vi "Find All Zeroes Inner Part (VI).vi"(6 "data":variant, 7 "f(x)":T1, 8 "error in":i32, 9 "accuracy":dbl=1e-08 format="%.2e", 10 "algorithm":u16, 11 "X and Y values":cluster{"X Values":dbl[], "Y Values":dbl[]} {"Y Values" format="%.2f"; "X Values" format="%.2f"}) -> (0 "error out":i32, 2 "f(Zeroes)":dbl[](array[numeric]) format="%.2f", 3 "Zeroes":dbl[](array[numeric]) format="%.2f")   [LabVIEW 2010, in "NI_Gmath.lvlib"]
uses:
  NI_Gmath.lvlib
  functionRefnum.ctl
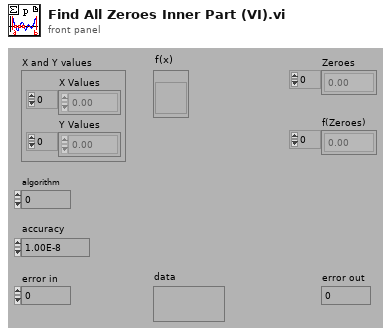
[diagram p1: front panel]
types:
  T1 = typedef "NI_Gmath.lvlib/functionRefnum.ctl" = refnum<vi>
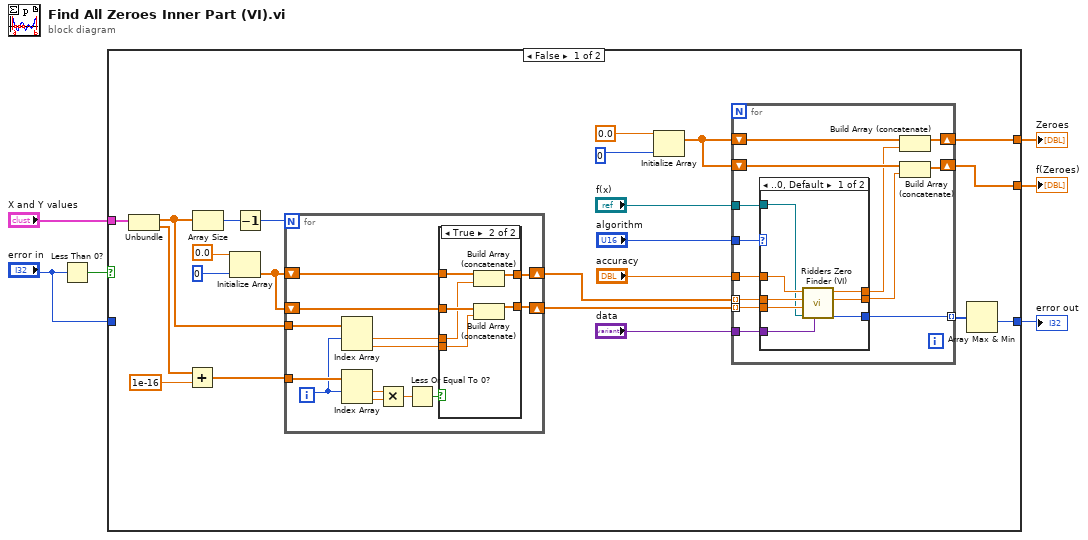
[diagram p0: block diagram]
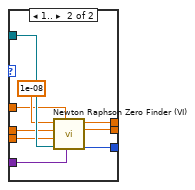
[diagram p2: hidden frame]
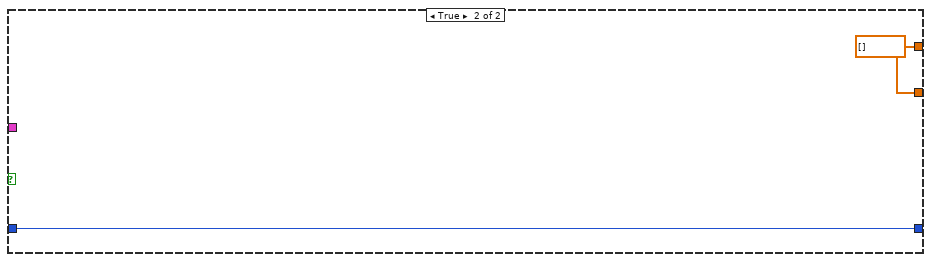
[diagram p4: hidden frame]
diagram:
  n1 = Less Than 0?(x="error in") -> (x < 0?=w2:bool)
  n2 = case shown="False" w2 {
    tunnel: "X and Y values" -> [w20 _]
    tunnel: [w11 w81] -> w5
    tunnel: [w10 w81] -> w4
    tunnel: [w9 w82] -> w3
    tunnel: "error in" -> [_ w82]
    frame False {
      n3 = Unbundle(w20) -> ("X Values"=w29:dbl[], "Y Values"=w23:dbl[])
      n4 = Add(x=w23, y=1e-16) -> (x+y=w25:dbl[])
      n5 = Array Size(array=w29) -> (size(s)=w21:i32)
      n6 = Initialize Array(0.0, 0) -> (w28:dbl[])
      n7 = Decrement(x=w21) -> (x-1=w22:i32)
      n8 = for {
        N: w22 -> [_]
        tunnel: w25 -> [w63]
        shift-right: [w69] -> w15
        shift-left: w28 -> [w70]
        shift-right: [w67] -> w14
        shift-left: w28 -> [w68]
        tunnel: w29 -> [w66]
        i -> [w60]
        n9 = Index Array(array=w66, index #1=w60) -> (element #1=w65:dbl, element #2=w64:dbl)  [unwired: 1 in]
        n10 = Index Array(array=w63, index #1=w60) -> (element #1=w62:dbl, element #2=w61:dbl)  [unwired: 1 in]
        n11 = Multiply(x=w62, y=w61) -> (x*y=w72:dbl)
        n12 = Less Or Equal To 0?(x=w72) -> (x <= 0?=w71:bool)
        n13 = case shown="True" w71 {
          tunnel: w70 -> [w74 w80]
          tunnel: [w74 w79] -> w69
          tunnel: w68 -> [w73 w78]
          tunnel: [w73 w77] -> w67
          tunnel: w65 -> [_ w76]
          tunnel: w64 -> [_ w75]
          frame False {
          }
          frame True {
            n14 = Build Array (concatenate)(w80, w76) -> (w79:dbl[])
            n15 = Build Array (concatenate)(w78, w75) -> (w77:dbl[])
          }
        }
      }
      n16 = Initialize Array(0.0, 0) -> (w18:dbl[])
      n17 = for {
        tunnel: w15 -> [w36] mode=indexing
        tunnel: w14 -> [w35] mode=indexing
        tunnel: "accuracy" -> [w34]
        shift-right: [w39] -> w11
        shift-left: w18 -> [w42]
        shift-right: [w40] -> w10
        shift-left: w18 -> [w41]
        tunnel: "algorithm" -> [w33]
        tunnel: [w32] -> w19 mode=indexing
        tunnel: "f(x)" -> [w31]
        tunnel: "data" -> [w30]
        n18 = case shown="..0, Default" w33 {
          tunnel: w34 -> [w50 w53]
          tunnel: w35 -> [w48 w51]
          tunnel: w36 -> [w49 w52]
          tunnel: [w45 w57] -> w37
          tunnel: [w46 w58] -> w38
          tunnel: [w47 w56] -> w32
          tunnel: w31 -> [w43 w55]
          tunnel: w30 -> [w44 w59]
          frame ..0, Default {
            n19 = call "Ridders Zero Finder (VI).vi"("data"=w44, "f(x)"=w43, "end"=w48, "start"=w49, "accuracy"=w50) -> ("error"=w47:i32, "f(zero)"=w45:dbl, "zero"=w46:dbl)  [unwired: 1 in, 3 out]
          }
          frame 1.. {
            n20 = call "Newton Raphson Zero Finder (VI).vi"("data"=w59, "accuracy"=w53, "f(x)"=w55, "end"=w51, "start"=w52, "h"=1e-08) -> ("error"=w56:i32, "f(zero)"=w57:dbl, "zero"=w58:dbl)  [unwired: 3 out]
          }
        }
        n21 = Build Array (concatenate)(w42, w38) -> (w39:dbl[])
        n22 = Build Array (concatenate)(w41, w37) -> (w40:dbl[])
      }
      n23 = Array Max & Min(array=w19) -> (min value=w9:i32)  [unwired: 3 out]
    }
    frame True {
      w81 = dbl[] []
    }
  }
  "error out" <- w3
  "f(Zeroes)" <- w4
  "Zeroes" <- w5
